vi "RequestFIFOMultiplexer.vi"   [LabVIEW 2016]
uses:
  <vilib>/rvi/Emulation/niFpgaGetClockAttributes.vi
  <vilib>/rvi/Emulation/niFpgaSctlEmulationGetInTimedLoop.vi
  <vilib>/rvi/Emulation/niFpgaEmulationReportErrorSimple.vi
  <vilib>/rvi/interface/RandomDataEmulation/niFpgaRandomDataHandleErrors.vi
  <vilib>/rvi/Emulation/niFpgaEmulationIsFPGAContextNoSignature.vi
  <vilib>/rvi/DataTransferAndStorage/Container/Common/niFpgaContainerGetUniqueNameForEmu.vi
  <vilib>/rvi/Memory/Memory_Emulation/niFpgaMemoryEmulationCacheClearOnFirstRun.vi
  <vilib>/rvi/Memory/Memory_Emulation/nirvimemoryEmulationManagerCache_MakeExclusive.vi
  <vilib>/rvi/Memory/Memory_Emulation/niFpgaMemoryEmulationValidateCache.vi
  <vilib>/rvi/Memory/Memory_Emulation/nirvimemoryEmulationManagerCache_InsertValue.vi
  <vilib>/Utility/error.llb/Clear Errors.vi
  <vilib>/rvi/Memory/Memory_Emulation/nirvimemoryEmulationManagerCache_ReleaseExclusive.vi
  <vilib>/rvi/Memory/Memory_Emulation/nirvimemoryEmulationManagerCache_GetValue.vi
  <vilib>/rvi/Memory/Memory_Emulation/nirvimemoryEmulationManagerCache_SetValue.vi
  <vilib>/rvi/Emulation/niFpgaProcessEmulError.vi
  <vilib>/rvi/eio/common/nirviEmuTemplateMethod_errors.vi
  <vilib>/rvi/Emulation/niFpgaCriticalErrorInLSC.vi
  <vilib>/rvi/DataTransferAndStorage/Container/XNode/niFpgaContainer.xnode
  <vilib>/rvi/interface/RandomDataEmulation/nirviRandomDataFpgaReadWriteTemplate.vi
  <vilib>/rvi/DataTransferAndStorage/Register/Emulation/niFpgaRegisterEmulation.vi
  <vilib>/eio/EIONode/EIONode.xnode
types:
  T1 = typedef "PortTypes.ctl" = enum8{"NA", "Slot1/AI0-AccelerometerAx", "Slot1/AI1-AccelerometerAz", "Slot1/AI2-AccelerometerBy", "Slot1/AI3-AccelerometerBz", "Slot2/AI0-AccelerometerCx", "Slot2/AI1-AccelerometerCz", "Slot2/AI2-AccelerometerDy", "Slot2/AI3-AccelerometerDz", "Slot3/DIO0-ModbusSubnetATx", "Slot3/DIO1-ModbusSubnetBTx", "Slot3/DIO2-ModbusSubnetCTx", "Slot3/DIO3-ModbusSubnetDTx", "Slot3/DIO4-ModbusSubnetARx", "Slot3/DIO5-ModbusSubnetBRx", "Slot3/DIO6-ModbusSubnetCRx", "Slot3/DIO7-ModbusSubnetDRx", "Slot4/DIO0-ModbusSubnetETx", "Slot4/DIO1-GyroTx", "Slot4/DIO2", "Slot4/DIO3", "Slot4/DIO4-ModbusSubnetERx", "Slot4/DIO5-GyroRx", "Slot4/DIO6", "Slot4/DIO7", "Slot5/DI0", "Slot5/DI1", "Slot5/DI2", "Slot5/DI3", "Slot5/DI4", "Slot5/DI5", "Slot5/DI6", "Slot5/DI7", "Slot5/DI8", "Slot5/DI9", "Slot5/DI10", "Slot5/DI11", "Slot5/DI12", "Slot5/DI13", "Slot5/DI14", "Slot5/DI15", "Slot5/DI16", "Slot5/DI17", "Slot5/DI18", "Slot5/DI19", "Slot5/DI20", "Slot5/DI21", "Slot5/DI22", "Slot5/DI23", "Slot5/DI24", "Slot5/DI25", "Slot5/DI26", "Slot5/DI27", "Slot5/DI28", "Slot5/DI29", "Slot5/DI30", "Slot5/DI31", "Slot6/CH0-HeartbeatToSafetyController", "Slot6/CH1-CriticalFaultToSafetyController", "Slot6/CH2-MirrorLoweringRaisingToSafetyController", "Slot6/CH3-MirrorParkedToSafetyController", "Slot6/CH4-AirSupplyValveControl", "Slot6/CH5-MirrorCellLightControl", "Slot6/CH6", "Slot6/CH7", "Slot7/CH0", "Slot7/CH1", "Slot7/CH2", "Slot7/CH3", "Slot7/CH4", "Slot7/CH5", "Slot7/CH6", "Slot7/CH7", "Slot8/Port1", "Slot8/Port2", "Slot8/Port3", "Slot8/Port4", "Undefined1", "Undefined2", "Undefined3", "Undefined4", "Undefined5", "Undefined6", "Undefined7", "Undefined8", "Undefined9", "Undefined10", "Undefined11", "Undefined12", "Undefined13", "Undefined14", "Undefined15", "Undefined16", "Undefined17", "Undefined18", "Undefined19", "Undefined20", "Undefined21", "Undefined22", "Undefined23", "Undefined24", "Undefined25", "Undefined26", "Undefined27", "Undefined28", "Undefined29", "Undefined30", "Undefined31", "Undefined32", "Undefined33", "Undefined34", "Undefined35", "Undefined36", "Undefined37", "Undefined38", "Undefined39", "Undefined40", "Undefined41", "Undefined42", "Undefined43", "Undefined44", "Undefined45", "Undefined46", "Undefined47", "Undefined48", "Undefined49", "Undefined50", "Undefined51", "Undefined52", "Undefined53", "Undefined54", "Undefined55", "Undefined56", "Undefined57", "Undefined58", "Undefined59", "Undefined60", "Undefined61", "Undefined62", "Undefined63", "Undefined64", "Undefined65", "Undefined66", "Undefined67", "Undefined68", "Undefined69", "Undefined70", "Undefined71", "Undefined72", "Undefined73", "Undefined74", "Undefined75", "Undefined76", "Undefined77", "Undefined78", "Undefined79", "Undefined80", "Undefined81", "Undefined82", "Undefined83", "Undefined84", "Undefined85", "Undefined86", "Undefined87", "Undefined88", "Undefined89", "Undefined90", "Undefined91", "Undefined92", "Undefined93", "Undefined94", "Undefined95", "Undefined96", "Undefined97", "Undefined98", "Undefined99", "Undefined100", "Undefined101", "Undefined102", "Undefined103", "Undefined104", "Undefined105", "Undefined106", "Undefined107", "Undefined108", "Undefined109", "Undefined110", "Undefined111", "Undefined112", "Undefined113", "Undefined114", "Undefined115", "Undefined116", "Undefined117", "Undefined118", "Undefined119", "Undefined120", "Undefined121", "Undefined122", "Undefined123", "Undefined124", "Undefined125", "Undefined126", "Undefined127", "Undefined128", "Undefined129", "Undefined130", "Undefined131", "Undefined132", "Undefined133", "Undefined134", "Undefined135", "Undefined136", "Undefined137", "Undefined138", "Undefined139", "Undefined140", "Undefined141", "Undefined142", "Undefined143", "Undefined144", "Undefined145", "Undefined146", "Undefined147", "Undefined148", "Undefined149", "Undefined150", "Undefined151", "Undefined152", "Undefined153", "Undefined154", "Undefined155", "Undefined156", "Undefined157", "Undefined158", "Undefined159", "Undefined160", "Undefined161", "Undefined162", "Undefined163", "Undefined164", "Undefined165", "Undefined166", "Undefined167", "Undefined168", "Undefined169", "Undefined170", "Undefined171", "Undefined172", "Undefined173", "Undefined174", "Undefined175", "ModbusSoftwareTrigger", "Accelerometers", "HealthAndStatus", "Timestamp"}
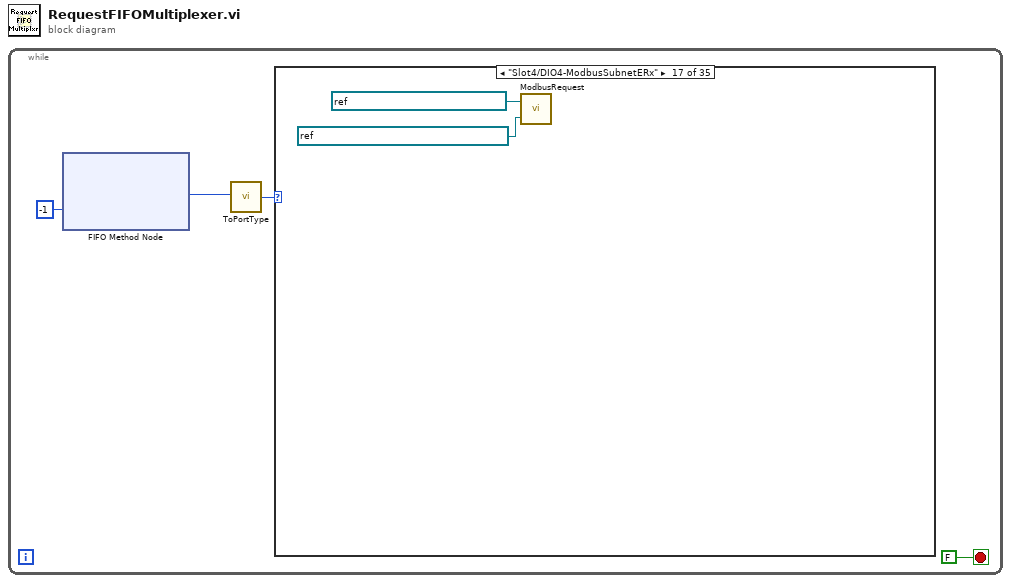
[diagram p0: block diagram]
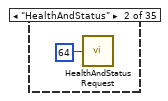
[diagram p3: hidden frame]
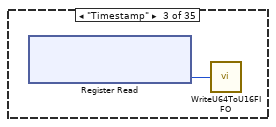
[diagram p4: hidden frame]
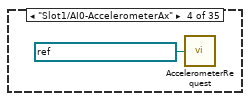
[diagram p5: hidden frame]
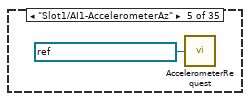
[diagram p6: hidden frame]
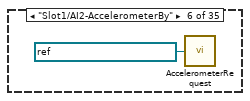
[diagram p7: hidden frame]
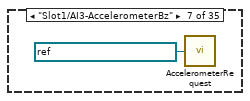
[diagram p8: hidden frame]
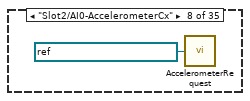
[diagram p9: hidden frame]
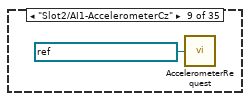
[diagram p10: hidden frame]
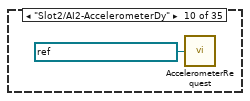
[diagram p11: hidden frame]
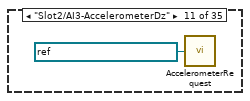
[diagram p12: hidden frame]
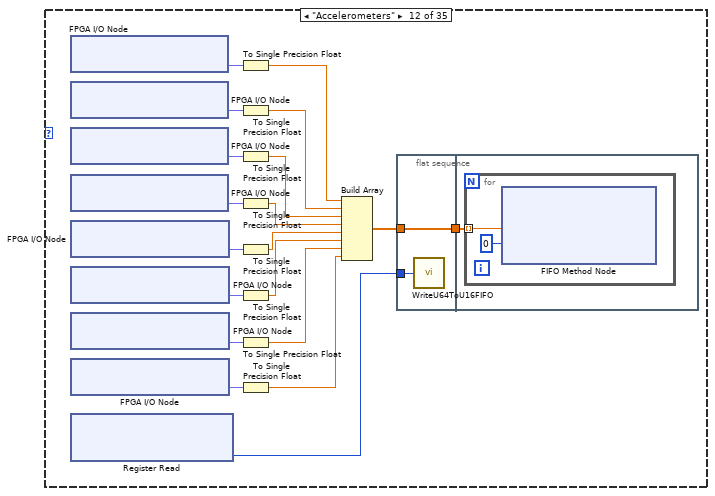
[diagram p13: hidden frame]
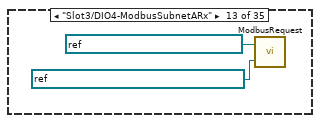
[diagram p14: hidden frame]
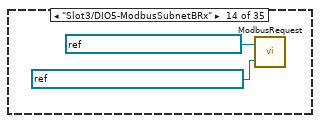
[diagram p15: hidden frame]
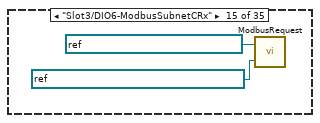
[diagram p16: hidden frame]
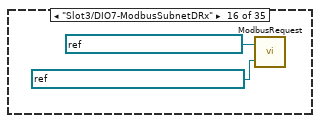
[diagram p17: hidden frame]
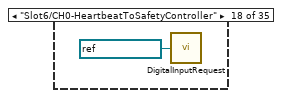
[diagram p18: hidden frame]
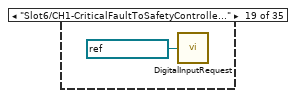
[diagram p19: hidden frame]
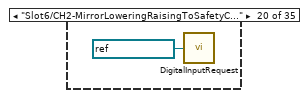
[diagram p20: hidden frame]
diagram:
  n1 = while {
    stop <- FALSE stop-if-true
    n2 = xnode ("FIFO Method Node")("Timeout"=-1) -> ("Element"=w3:u16)  [unwired: 1 in, 2 out]
    n3 = call "ToPortType.vi"("Input"=w3) -> ("PortTypes"=w2:T1)
    n4 = case shown="\"Slot4/DIO4-ModbusSubnetERx\"" w2 {
      frame "NA", Default {
      }
      frame "HealthAndStatus" {
        n5 = call "HealthAndStatusRequest.vi"("HealthAndStatusSize"=u32 64) -> ()  [unwired: 1 in]
      }
      frame "Timestamp" {
        n6 = xnode ("Register Read")() -> ("Data"=w6:u64)  [unwired: 1 in, 1 out]
        n7 = call "WriteU64ToU16FIFO.vi"("U64"=w6) -> ()  [unwired: 1 in]
      }
      frame "Slot1/AI0-AccelerometerAx" {
        n8 = call "AccelerometerRequest.vi"("FPGA I/O In"=refnum<k21> "AccelerometerAB/AI0") -> ()  [unwired: 1 in]
      }
      frame "Slot1/AI1-AccelerometerAz" {
        n9 = call "AccelerometerRequest.vi"("FPGA I/O In"=refnum<k21> "AccelerometerAB/AI1") -> ()  [unwired: 1 in]
      }
      frame "Slot1/AI2-AccelerometerBy" {
        n10 = call "AccelerometerRequest.vi"("FPGA I/O In"=refnum<k21> "AccelerometerAB/AI2") -> ()  [unwired: 1 in]
      }
      frame "Slot1/AI3-AccelerometerBz" {
        n11 = call "AccelerometerRequest.vi"("FPGA I/O In"=refnum<k21> "AccelerometerAB/AI3") -> ()  [unwired: 1 in]
      }
      frame "Slot2/AI0-AccelerometerCx" {
        n12 = call "AccelerometerRequest.vi"("FPGA I/O In"=refnum<k21> "AccelerometerCD/AI0") -> ()  [unwired: 1 in]
      }
      frame "Slot2/AI1-AccelerometerCz" {
        n13 = call "AccelerometerRequest.vi"("FPGA I/O In"=refnum<k21> "AccelerometerCD/AI1") -> ()  [unwired: 1 in]
      }
      frame "Slot2/AI2-AccelerometerDy" {
        n14 = call "AccelerometerRequest.vi"("FPGA I/O In"=refnum<k21> "AccelerometerCD/AI2") -> ()  [unwired: 1 in]
      }
      frame "Slot2/AI3-AccelerometerDz" {
        n15 = call "AccelerometerRequest.vi"("FPGA I/O In"=refnum<k21> "AccelerometerCD/AI3") -> ()  [unwired: 1 in]
      }
      frame "Accelerometers" {
        n16 = xnode "FPGA I/O Node"() -> ("AccelerometerAB/AI0"=w26:fxp<+/-,24,5>)  [unwired: 1 in, 1 out]
        n17 = xnode "FPGA I/O Node"() -> ("AccelerometerAB/AI1"=w27:fxp<+/-,24,5>)  [unwired: 1 in, 1 out]
        n18 = xnode "FPGA I/O Node"() -> ("AccelerometerAB/AI2"=w28:fxp<+/-,24,5>)  [unwired: 1 in, 1 out]
        n19 = xnode "FPGA I/O Node"() -> ("AccelerometerAB/AI3"=w29:fxp<+/-,24,5>)  [unwired: 1 in, 1 out]
        n20 = xnode "FPGA I/O Node"() -> ("AccelerometerCD/AI0"=w30:fxp<+/-,24,5>)  [unwired: 1 in, 1 out]
        n21 = xnode "FPGA I/O Node"() -> ("AccelerometerCD/AI1"=w31:fxp<+/-,24,5>)  [unwired: 1 in, 1 out]
        n22 = xnode "FPGA I/O Node"() -> ("AccelerometerCD/AI2"=w32:fxp<+/-,24,5>)  [unwired: 1 in, 1 out]
        n23 = xnode "FPGA I/O Node"() -> ("AccelerometerCD/AI3"=w33:fxp<+/-,24,5>)  [unwired: 1 in, 1 out]
        n24 = xnode ("Register Read")() -> ("Data"=w15:u64)  [unwired: 1 in, 1 out]
        n25 = To Single Precision Float(number=w26) -> (single precision float=w25:sgl)
        n26 = To Single Precision Float(number=w27) -> (single precision float=w24:sgl)
        n27 = To Single Precision Float(number=w28) -> (single precision float=w23:sgl)
        n28 = To Single Precision Float(number=w29) -> (single precision float=w22:sgl)
        n29 = To Single Precision Float(number=w30) -> (single precision float=w18:sgl)
        n30 = To Single Precision Float(number=w31) -> (single precision float=w19:sgl)
        n31 = To Single Precision Float(number=w32) -> (single precision float=w20:sgl)
        n32 = To Single Precision Float(number=w33) -> (single precision float=w21:sgl)
        n33 = Build Array(w25, w24, w23, w22, w18, w19, w20, w21) -> (w17:sgl[])
        n34 = flat-sequence {
          tunnel: w17 -> [w35]
          tunnel: [w35] -> w16
          tunnel: w15 -> [w34]
          tunnel: w16 -> [w36]
          frame #0 {
            n35 = call "WriteU64ToU16FIFO.vi"("U64"=w34) -> ()  [unwired: 1 in]
          }
          frame #1 {
            n36 = for {
              tunnel: w36 -> [w38] mode=indexing
              n37 = xnode ("FIFO Method Node")("Element"=w38, "Timeout"=0) -> ()  [unwired: 1 in, 2 out]
            }
          }
        }
      }
      frame "Slot3/DIO4-ModbusSubnetARx" {
        n38 = call "ModbusRequest.vi"("ModbusSubnetTimestampFIFO"=refnum<k21> "ModbusSubnetATxTimestampFIFO", "ModbusSubnetRxFIFO"=refnum<k21> "ModbusSubnetARxDataFIFO") -> ()  [unwired: 1 in]
      }
      frame "Slot3/DIO5-ModbusSubnetBRx" {
        n39 = call "ModbusRequest.vi"("ModbusSubnetTimestampFIFO"=refnum<k21> "ModbusSubnetBTxTimestampFIFO", "ModbusSubnetRxFIFO"=refnum<k21> "ModbusSubnetBRxDataFIFO") -> ()  [unwired: 1 in]
      }
      frame "Slot3/DIO6-ModbusSubnetCRx" {
        n40 = call "ModbusRequest.vi"("ModbusSubnetTimestampFIFO"=refnum<k21> "ModbusSubnetCTxTimestampFIFO", "ModbusSubnetRxFIFO"=refnum<k21> "ModbusSubnetCRxDataFIFO") -> ()  [unwired: 1 in]
      }
      frame "Slot3/DIO7-ModbusSubnetDRx" {
        n41 = call "ModbusRequest.vi"("ModbusSubnetTimestampFIFO"=refnum<k21> "ModbusSubnetDTxTimestampFIFO", "ModbusSubnetRxFIFO"=refnum<k21> "ModbusSubnetDRxDataFIFO") -> ()  [unwired: 1 in]
      }
      frame "Slot4/DIO4-ModbusSubnetERx" {
        n42 = call "ModbusRequest.vi"("ModbusSubnetTimestampFIFO"=refnum<k21> "ModbusSubnetETxTimestampFIFO", "ModbusSubnetRxFIFO"=refnum<k21> "ModbusSubnetERxDataFIFO") -> ()  [unwired: 1 in]
      }
      frame "Slot6/CH0-HeartbeatToSafetyController" {
        n43 = call "DigitalInputRequest.vi"("FPGA I/O In"=refnum<k21> "Slot6/CH0") -> ()  [unwired: 1 in]
      }
      frame "Slot6/CH1-CriticalFaultToSafetyController" {
        n44 = call "DigitalInputRequest.vi"("FPGA I/O In"=refnum<k21> "Slot6/CH1") -> ()  [unwired: 1 in]
      }
      frame "Slot6/CH2-MirrorLoweringRaisingToSafetyController" {
        n45 = call "DigitalInputRequest.vi"("FPGA I/O In"=refnum<k21> "Slot6/CH2") -> ()  [unwired: 1 in]
      }
      frame "Slot6/CH3-MirrorParkedToSafetyController" {
        n46 = call "DigitalInputRequest.vi"("FPGA I/O In"=refnum<k21> "Slot6/CH3") -> ()  [unwired: 1 in]
      }
      frame "Slot6/CH4-AirSupplyValveControl" {
        n47 = call "DigitalInputRequest.vi"("FPGA I/O In"=refnum<k21> "Slot6/CH4") -> ()  [unwired: 1 in]
      }
      frame "Slot6/CH5-MirrorCellLightControl" {
        n48 = call "DigitalInputRequest.vi"("FPGA I/O In"=refnum<k21> "Slot6/CH5") -> ()  [unwired: 1 in]
      }
      frame "Slot6/CH6" {
        n49 = call "DigitalInputRequest.vi"("FPGA I/O In"=refnum<k21> "Slot6/CH6") -> ()  [unwired: 1 in]
      }
      frame "Slot6/CH7" {
        n50 = call "DigitalInputRequest.vi"("FPGA I/O In"=refnum<k21> "Slot6/CH7") -> ()  [unwired: 1 in]
      }
      frame "Slot7/CH0" {
        n51 = call "DigitalInputRequest.vi"("FPGA I/O In"=refnum<k21> "Slot7/CH0") -> ()  [unwired: 1 in]
      }
      frame "Slot7/CH1" {
        n52 = call "DigitalInputRequest.vi"("FPGA I/O In"=refnum<k21> "Slot7/CH1") -> ()  [unwired: 1 in]
      }
      frame "Slot7/CH2" {
        n53 = call "DigitalInputRequest.vi"("FPGA I/O In"=refnum<k21> "Slot7/CH2") -> ()  [unwired: 1 in]
      }
      frame "Slot7/CH3" {
        n54 = call "DigitalInputRequest.vi"("FPGA I/O In"=refnum<k21> "Slot7/CH3") -> ()  [unwired: 1 in]
      }
      frame "Slot7/CH4" {
        n55 = call "DigitalInputRequest.vi"("FPGA I/O In"=refnum<k21> "Slot7/CH4") -> ()  [unwired: 1 in]
      }
      frame "Slot7/CH5" {
        n56 = call "DigitalInputRequest.vi"("FPGA I/O In"=refnum<k21> "Slot7/CH5") -> ()  [unwired: 1 in]
      }
      frame "Slot7/CH6" {
        n57 = call "DigitalInputRequest.vi"("FPGA I/O In"=refnum<k21> "Slot7/CH6") -> ()  [unwired: 1 in]
      }
      frame "Slot7/CH7" {
        n58 = call "DigitalInputRequest.vi"("FPGA I/O In"=refnum<k21> "Slot7/CH7") -> ()  [unwired: 1 in]
      }
      frame "Slot8/Port1" {
        n59 = call "RS232Request.vi"("InputFIFO"=refnum<k21> "DisplacementRxFIFO") -> ()  [unwired: 1 in]
      }
      frame "Slot8/Port2" {
        n60 = call "RS232Request.vi"("InputFIFO"=refnum<k21> "InclinometerRxFIFO") -> ()  [unwired: 1 in]
      }
    }
  }
